vi "load RT config file.vi"(11 "configuration file path (RT local)":path) -> (0 "error out":errorcluster, 1 "unmatched parameters":string[](array[string]), 2 "Default parameters":string[](array[string]), 3 "config data out":T18={"Message"={"Parameters"={"FPGA Ref"=refnum, "configID"=0, "activeChannels"=[]}, "Variables"={"RT Status"={"Comms loop"=FALSE, "scheduler loop"=FALSE, "data process loop"=FALSE, "FIFO loop"=FALSE, "Command Stream"=FALSE, "Error Stream"=FALSE, "FPGA FIFO"=FALSE, "Data Stream"=FALSE}, "watchdog"=timestamp(0 s since 1904-01-01), "limitsEnabled"=FALSE, "Interlocks"={"gearboxOil"=FALSE, "bearingOil"=FALSE, "gearboxAir"=FALSE}}}, "FIFO"={"Params"={"FPGA ref"=refnum, "Total Channels"=0}, "Variables"={"FIFO wait counter"=0, "FIFO read trigger"=0}}, "Comms data"={"Parameters"={"error writer name"="", "command reader name"="", "error buffer size"=0, "command buffer size"=0, "scanivalveIP"="", "scanivalvePeriod"=0}, "Variables"={"listen schedule"=0, "incident buffer"=[], "command stream"="", "error stream"="", "waiting for command stream connect"=FALSE, "waiting for error stream connect"=FALSE, "scanivalve connection"=refnum, "scanivalveScheduleID"=0, "activeScanivalvePorts"=[], "channelCount"=0}, "scanivalveConfig"={"listS"={"period"=0, "ADtrig"=FALSE, "ScanTrig"=FALSE, "page"=0, "qpkts"=0}, "listC"={"ZC"=FALSE, "unitScan"="", "CvtUnit"=0.0, "bin"=FALSE, "EU"=FALSE}, "listSG"={"Avg1"=0, "FPS1"=0, "SGEnable1"=FALSE}, "activeChannels"={"Chan1"={"101"=FALSE, "102"=FALSE, "103"=FALSE, "104"=FALSE, "109"=FALSE, "110"=FALSE, "111"=FALSE, "112"=FALSE, "201"=FALSE, "202"=FALSE, "203"=FALSE, "204"=FALSE, "209"=FALSE, "210"=FALSE, "211"=FALSE, "212"=FALSE, "301"=FALSE, "302"=FALSE, "303"=FALSE, "304"=FALSE, "309"=FALSE, "310"=FALSE, "311"=FALSE, "312"=FALSE, "401"=FALSE, "402"=FALSE, "403"=FALSE, "404"=FALSE, "409"=FALSE, "410"=FALSE, "411"=FALSE, "412"=FALSE}}}}, "Data processor"={"Parameters"={"FPGA Ref"=refnum, "data stream"={"data writer name"="error writer", "NS write buffer size"=16, "NS Buffer length"=0}, "FIFO Depth"=0, "Channel controls"={"FIFO channel count"=0, "active indices"=[], "active channels"=0, "channelScaling"=[], "scanivalveCount"=0, "channels"=[]}, "safetyChannels"={"oilP"=0, "airP"=0, "water"=0, "channelLimits"=[]}, "speedChannel"=0, "maxSpeedLimit"=0.0, "Torque"={"fixedOffset"=0.0, "filter"=FALSE, "fallingEdge"=FALSE, "swapEncoders"=FALSE}}, "Variables"={"Intermediary buffer"=[], "buffer position"=0, "write loop counter"=0, "NS write trigger"=0, "NS Connection status"=FALSE, "waiting for NS"=FALSE, "labAmbient"={"pressure"=0.0, "temperature"=0.0}, "scanivalvePorts"=[], "scanivalvePressures"=[], "data stream"="", "activeChannelLimitIndex"=[], "runningSpeedLimit"=0.0, "speedChannelIndex"=0, "Interlocks"={"gearboxOil"=FALSE, "bearingOil"=FALSE, "gearboxAir"=FALSE}, "interlockChannels"={"gearboxOil"=0, "bearingOil"=0, "air"=0}, "limitStates"=[]}}})   [LabVIEW 2018]
uses:
  RT/Type Defs/Message loop data.ctl
  RT/Type Defs/FPGA reference.ctl
  RT/Type Defs/RT Status.ctl
  RT/Type Defs/Analogue loop data.ctl
  RT/Communications loop/comms data.ctl
  RT/Type Defs/generic incident.ctl
  ICL-LabVIEW_General/Scanivalve API project/full interface/polymorphic/scanivalveConfig.ctl
  ICL-LabVIEW_General/Scanivalve API project/full interface/listS.ctl
  ICL-LabVIEW_General/Scanivalve API project/full interface/listC.ctl
  ICL-LabVIEW_General/Scanivalve API project/full interface/listSG.ctl
  ICL-LabVIEW_General/Scanivalve API project/full interface/chan1.ctl
  RT/Type Defs/Data processing loop data.ctl
  type defs/channelControl.ctl
  RT/Type Defs/channelScalingTypes.ctl
  RT/Type Defs/scalingMethods.ctl
  ICL-LabVIEW_General/data channels/parent class/Data Channel.lvclass
  type defs/channelLimitControl.ctl
  type defs/limitActions.ctl
  RT/Type Defs/configFilePath.ctl
  <vilib>/Utility/config.llb/Read Key (U32).vi
  <vilib>/Utility/config.llb/Read Key (String).vi
  <vilib>/Utility/config.llb/Read Key (I32).vi
  <vilib>/Utility/config.llb/Read Key (Double).vi
  <vilib>/Utility/config.llb/Read Key (Boolean).vi
  <vilib>/Utility/config.llb/NI_LVConfig.lvlib
  ICL-LabVIEW_General/Scanivalve API project/Scanivalve API.lvlib
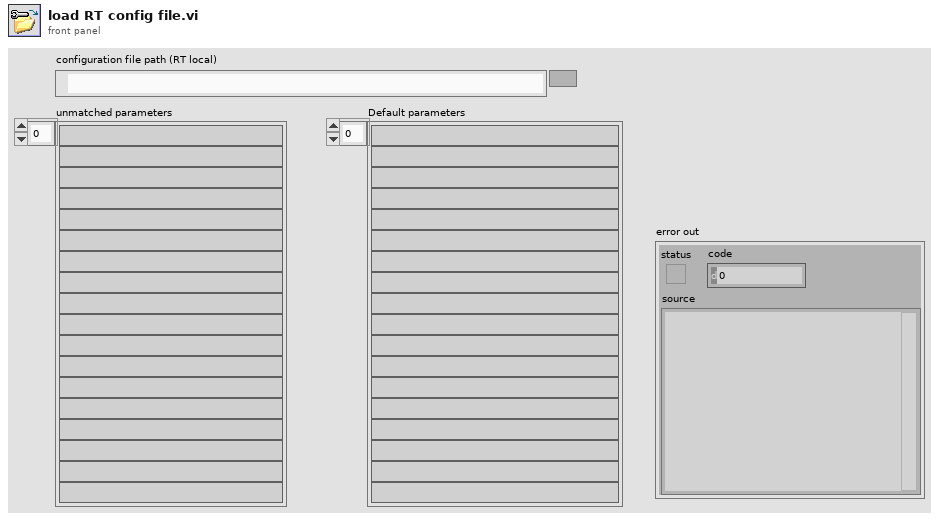
[diagram p1: front panel]
types:
  T1 = typedef "Message loop data.ctl" = cluster{"Parameters":cluster{"FPGA Ref":T2, "configID":u32, "activeChannels":cluster{"index":u16, "name":string}[]}, "Variables":cluster{"RT Status":T3, "watchdog":timestamp, "limitsEnabled":bool, "Interlocks":cluster{"gearboxOil":bool, "bearingOil":bool, "gearboxAir":bool}}}
  T2 = typedef "FPGA reference.ctl" = refnum<k20>
  T3 = typedef "RT Status.ctl" = cluster{"Comms loop":bool, "scheduler loop":bool, "data process loop":bool, "FIFO loop":bool, "Command Stream":bool, "Error Stream":bool, "FPGA FIFO":bool, "Data Stream":bool}
  T4 = typedef "Analogue loop data.ctl" = cluster{"Params":cluster{"FPGA ref":T2, "Total Channels":u32}, "Variables":cluster{"FIFO wait counter":u16, "FIFO read trigger":u32}}
  T5 = typedef "comms data.ctl" = cluster{"Parameters":cluster{"error writer name":string, "command reader name":string, "error buffer size":i32, "command buffer size":i32, "scanivalveIP":string, "scanivalvePeriod":u16}, "Variables":cluster{"listen schedule":u32, "incident buffer":T6[], "command stream":refnum<k21>, "error stream":refnum<k21>, "waiting for command stream connect":bool, "waiting for error stream connect":bool, "scanivalve connection":refnum<k5>, "scanivalveScheduleID":u32, "activeScanivalvePorts":i32[], "channelCount":i16}, "scanivalveConfig":T7}
  T6 = typedef "generic incident.ctl" = cluster{"timestamp":timestamp, "type":string, "Variant":variant}
  T7 = typedef "Scanivalve API.lvlib/scanivalveConfig.ctl" = cluster{"listS":T8, "listC":T9, "listSG":T10, "activeChannels":T11}
  T8 = typedef "Scanivalve API.lvlib/listS.ctl" = cluster{"period":u16, "ADtrig":bool, "ScanTrig":bool, "page":u16, "qpkts":u16}
  T9 = typedef "Scanivalve API.lvlib/listC.ctl" = cluster{"ZC":bool, "unitScan":string, "CvtUnit":dbl, "bin":bool, "EU":bool}
  T10 = typedef "Scanivalve API.lvlib/listSG.ctl" = cluster{"Avg1":u16, "FPS1":u16, "SGEnable1":bool}
  T11 = typedef "Scanivalve API.lvlib/chan1.ctl" = cluster{"Chan1":cluster{"101":bool, "102":bool, "103":bool, "104":bool, "109":bool, "110":bool, "111":bool, "112":bool, "201":bool, "202":bool, "203":bool, "204":bool, "209":bool, "210":bool, "211":bool, "212":bool, "301":bool, "302":bool, "303":bool, "304":bool, "309":bool, "310":bool, "311":bool, "312":bool, "401":bool, "402":bool, "403":bool, "404":bool, "409":bool, "410":bool, "411":bool, "412":bool}}
  T12 = typedef "Data processing loop data.ctl" = cluster{"Parameters":cluster{"FPGA Ref":T2, "data stream":cluster{"data writer name":string, "NS write buffer size":i32, "NS Buffer length":u32}, "FIFO Depth":u32, "Channel controls":cluster{"FIFO channel count":i32, "active indices":i16[], "active channels":i32, "channelScaling":T13[], "scanivalveCount":i32, "channels":refnum<class "Data Channel.lvclass">[]}, "safetyChannels":cluster{"oilP":u16, "airP":u16, "water":u16, "channelLimits":T16[]}, "speedChannel":i32, "maxSpeedLimit":dbl, "Torque":cluster{"fixedOffset":dbl, "filter":bool, "fallingEdge":bool, "swapEncoders":bool}}, "Variables":cluster{"Intermediary buffer":dbl[][], "buffer position":u32, "write loop counter":u16, "NS write trigger":u32, "NS Connection status":bool, "waiting for NS":bool, "labAmbient":cluster{"pressure":dbl, "temperature":dbl}, "scanivalvePorts":u16[], "scanivalvePressures":dbl[], "data stream":refnum<k21>, "activeChannelLimitIndex":u16[], "runningSpeedLimit":dbl, "speedChannelIndex":i32, "Interlocks":cluster{"gearboxOil":bool, "bearingOil":bool, "gearboxAir":bool}, "interlockChannels":cluster{"gearboxOil":i32, "bearingOil":i32, "air":i32}, "limitStates":cluster{"warn":bool, "alarm":bool}[]}}
  T13 = typedef "channelControl.ctl" = cluster{"index":u16, "active":bool, "channelType":T14, "module":u16, "terminal":u16, "channelName":string, "scalingMethod":T15, "scalingParameters":dbl[], "scaledUnits":string, "tempOffset":dbl}
  T14 = typedef "channelScalingTypes.ctl" = enum16{"calculation", "measurement", "scanivalve", "output", "digital"}
  T15 = typedef "scalingMethods.ctl" = enum16{"none", "linear", "thermocouple", "polynomial", "encoder", "RTD"}
  T16 = typedef "channelLimitControl.ctl" = cluster{"channelID":u16, "Enabled":bool, "warnValue":dbl, "limitValue":dbl, "Invert":bool, "limitAction":T17}
  T17 = typedef "limitActions.ctl" = enum16{"stop", "shutdown", "ignore"}
  T18 = cluster{"Message":T1, "FIFO":T4, "Comms data":T5, "Data processor":T12}
  T19 = typedef "configFilePath.ctl" = path
  T20 = typedef "NI_LVConfig.lvlib/Config Data RefNum.ctl" = refnum<k1>
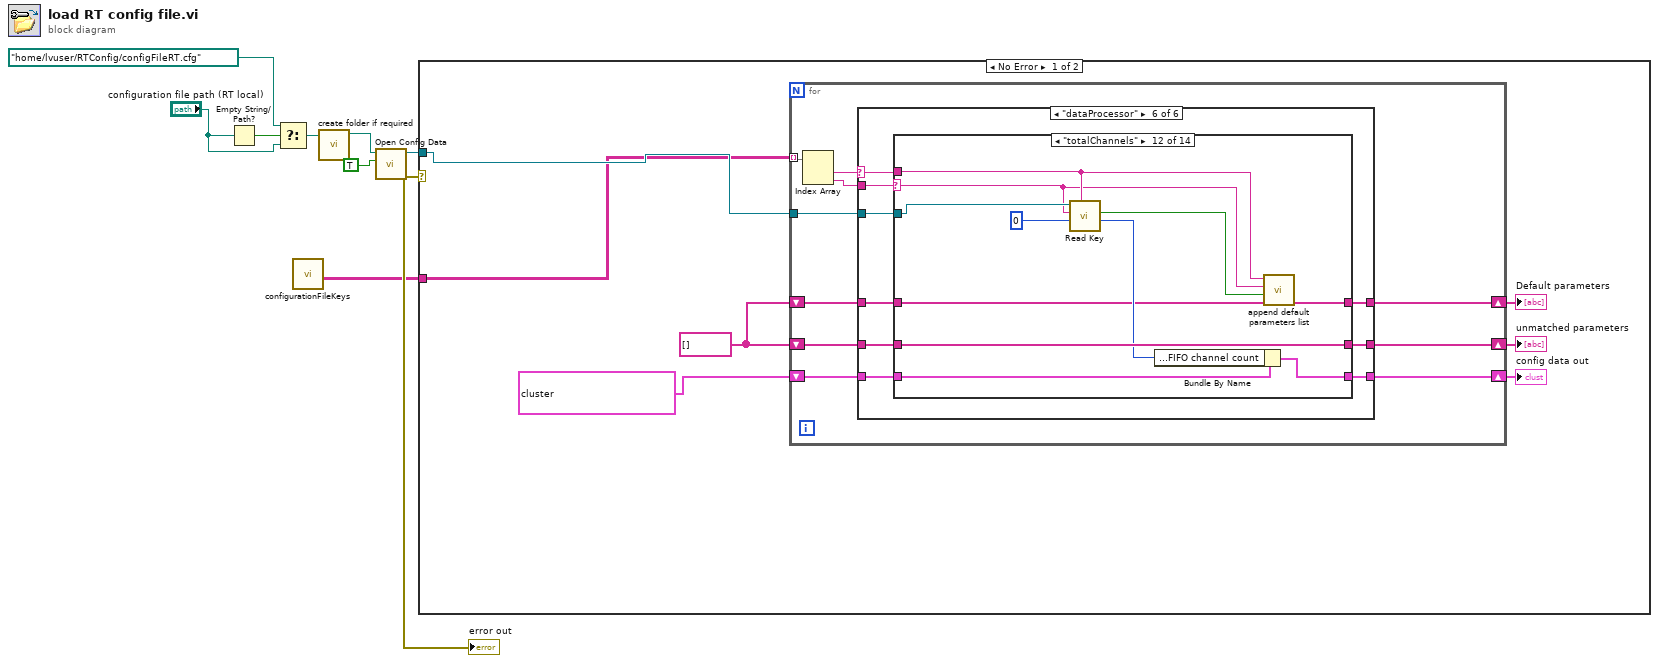
[diagram p0: block diagram]
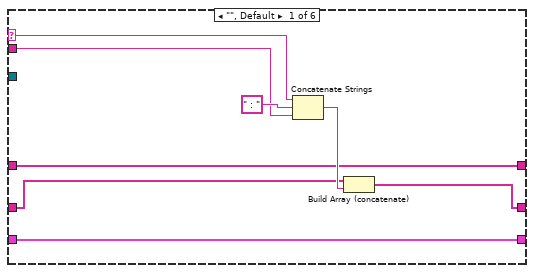
[diagram p2: hidden frame]
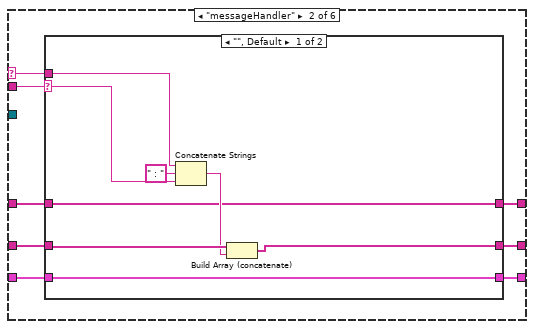
[diagram p3: hidden frame]
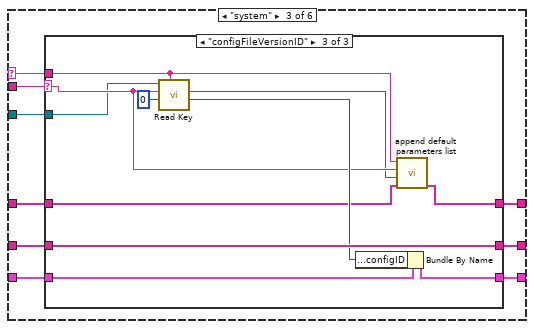
[diagram p5: hidden frame]
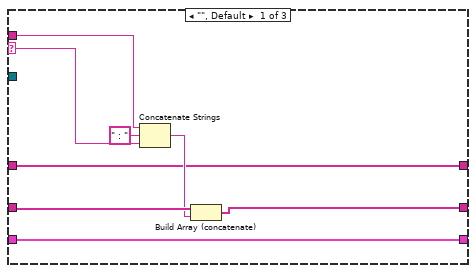
[diagram p6: hidden frame]
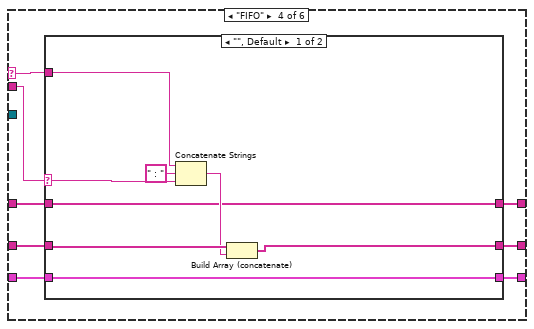
[diagram p8: hidden frame]
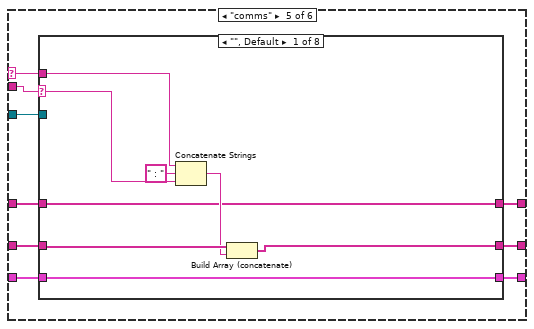
[diagram p10: hidden frame]
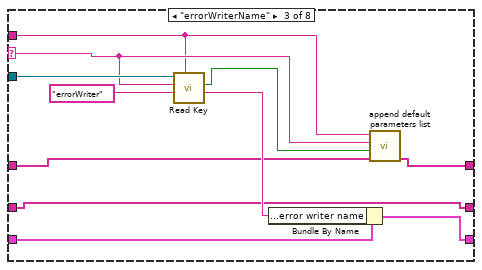
[diagram p12: hidden frame]
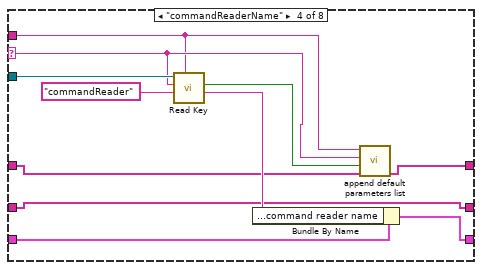
[diagram p13: hidden frame]
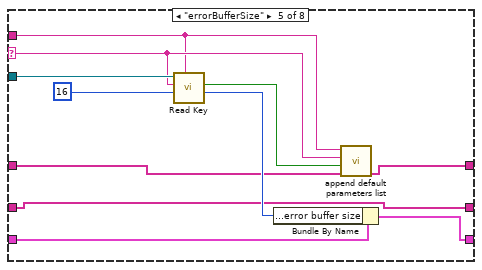
[diagram p14: hidden frame]
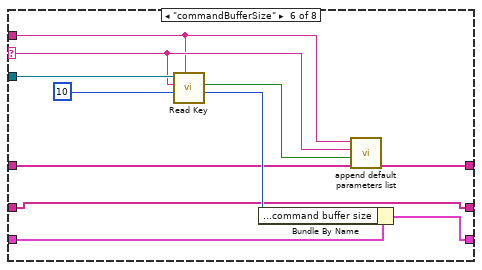
[diagram p15: hidden frame]
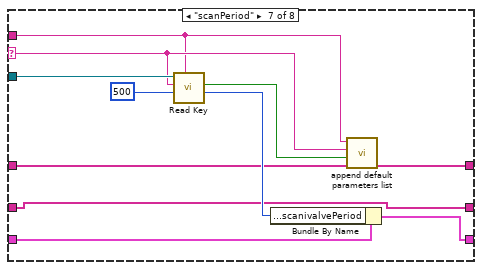
[diagram p16: hidden frame]
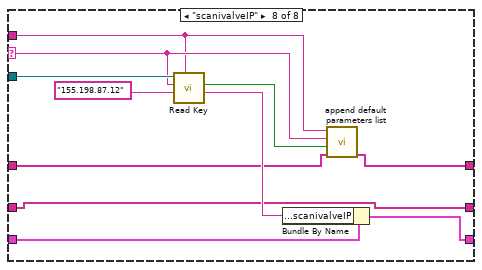
[diagram p17: hidden frame]
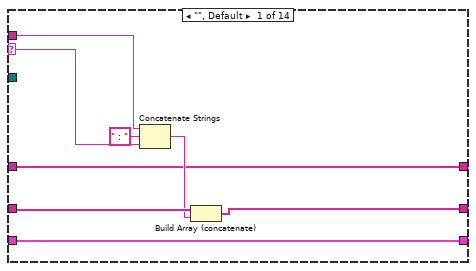
[diagram p18: hidden frame]
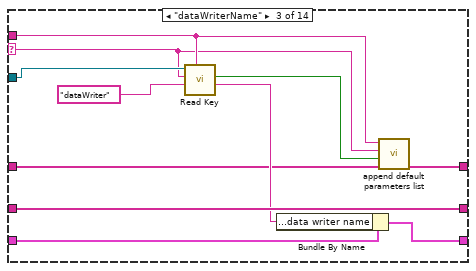
[diagram p20: hidden frame]
diagram:
  n1 = Empty String/Path?(string/path="configuration file path (RT local)") -> (empty?=w6:bool)
  n2 = Select(t=T19 path "/home/lvuser/RTConfig/configFileRT.cfg" ("file path (use dialog)"), s=w6, f="configuration file path (RT local)") -> (s? t:f=w2:T19)
  n3 = call "configurationFileKeys.vi"() -> ("configKeysRT"=w4:string[][])  [unwired: 9 in, 2 out]
  n4 = call "create folder if required.vi"("folder path"=w2) -> ("actual path"=w1:path)  [unwired: 9 in, 1 out]
  n5 = call <vilib>:"Open Config Data.vi"("create file if necessary (T)"=TRUE, "configuration file path"=w1) -> ("error out"=w7:errorcluster, "refnum"=w9:T20)  [unwired: 7 in, 1 out]
  "error out" <- w7
  n6 = case shown="No Error" w7 {
    tunnel: w9 -> [w14 _]
    tunnel: w4 -> [w13 _]
    frame No Error {
      w12 = string[] []
      n7 = for {
        shift-right: [w25] -> w16
        shift-left: w12 -> [w26]
        shift-right: [w23] -> w10
        shift-left: T18 {"Message"={"Parameters"={"FPGA Ref"=refnum, "configID"=0, "activeChannels"=[]}, "Variables"={"RT Status"={"Comms loop"=FALSE, "scheduler loop"=FALSE, "data process loop"=FALSE, "FIFO loop"=FALSE, "Command Stream"=FALSE, "Error Stream"=FALSE, "FPGA FIFO"=FALSE, "Data Stream"=FALSE}, "watchdog"=timestamp(0 s since 1904-01-01), "limitsEnabled"=FALSE, "Interlocks"={"gearboxOil"=FALSE, "bearingOil"=FALSE, "gearboxAir"=FALSE}}}, "FIFO"={"Params"={"FPGA ref"=refnum, "Total Channels"=0}, "Variables"={"FIFO wait counter"=0, "FIFO read trigger"=0}}, "Comms data"={"Parameters"={"error writer name"="error writer", "command reader name"="command reader", "error buffer size"=16, "command buffer size"=16, "scanivalveIP"="", "scanivalvePeriod"=16}, "Variables"={"listen schedule"=0, "incident buffer"=[], "command stream"="", "error stream"="", "waiting for command stream connect"=FALSE, "waiting for error stream connect"=FALSE, "scanivalve connection"=refnum, "scanivalveScheduleID"=16, "activeScanivalvePorts"=[], "channelCount"=0}, "scanivalveConfig"={"listS"={"period"=0, "ADtrig"=FALSE, "ScanTrig"=FALSE, "page"=0, "qpkts"=0}, "listC"={"ZC"=FALSE, "unitScan"="", "CvtUnit"=0.0, "bin"=FALSE, "EU"=FALSE}, "listSG"={"Avg1"=0, "FPS1"=0, "SGEnable1"=FALSE}, "activeChannels"={"Chan1"={"101"=FALSE, "102"=FALSE, "103"=FALSE, "104"=FALSE, "109"=FALSE, "110"=FALSE, "111"=FALSE, "112"=FALSE, "201"=FALSE, "202"=FALSE, "203"=FALSE, "204"=FALSE, "209"=FALSE, "210"=FALSE, "211"=FALSE, "212"=FALSE, "301"=FALSE, "302"=FALSE, "303"=FALSE, "304"=FALSE, "309"=FALSE, "310"=FALSE, "311"=FALSE, "312"=FALSE, "401"=FALSE, "402"=FALSE, "403"=FALSE, "404"=FALSE, "409"=FALSE, "410"=FALSE, "411"=FALSE, "412"=FALSE}}}}, "Data processor"={"Parameters"={"FPGA Ref"=refnum, "data stream"={"data writer name"="", "NS write buffer size"=0, "NS Buffer length"=0}, "FIFO Depth"=0, "Channel controls"={"FIFO channel count"=0, "active indices"=[], "active channels"=0, "channelScaling"=[], "scanivalveCount"=0, "channels"=[]}, "safetyChannels"={"oilP"=0, "airP"=0, "water"=0, "channelLimits"=[]}, "speedChannel"=0, "maxSpeedLimit"=0.0, "Torque"={"fixedOffset"=0.0, "filter"=FALSE, "fallingEdge"=FALSE, "swapEncoders"=FALSE}}, "Variables"={"Intermediary buffer"=[], "buffer position"=0, "write loop counter"=0, "NS write trigger"=0, "NS Connection status"=FALSE, "waiting for NS"=FALSE, "labAmbient"={"pressure"=0.0, "temperature"=0.0}, "scanivalvePorts"=[], "scanivalvePressures"=[], "data stream"="", "activeChannelLimitIndex"=[], "runningSpeedLimit"=0.0, "speedChannelIndex"=0, "Interlocks"={"gearboxOil"=FALSE, "bearingOil"=FALSE, "gearboxAir"=FALSE}, "interlockChannels"={"gearboxOil"=0, "bearingOil"=0, "air"=0}, "limitStates"=[]}}} ("config data 2") -> [w24]
        tunnel: w14 -> [w22]
        tunnel: w13 -> [w21] mode=indexing
        shift-right: [w18] -> w11
        shift-left: w12 -> [w17]
        n8 = Index Array(array=w21) -> (element #1=w20:string, element #2=w19:string)  [unwired: 2 in]
        n9 = case shown="\"dataProcessor\"" w20 {
          selector: w20 -> [w30 w41 w61 w91 w111 w197]
          tunnel: w26 -> [w32 w42 w62 w92 w112 w198]
          tunnel: [w31 w40 w60 w90 w110 w196] -> w25
          tunnel: w24 -> [w29 w38 w58 w88 w109 w194]
          tunnel: [w29 w39 w59 w89 w108 w195] -> w23
          tunnel: w22 -> [_ _ w54 _ w107 w193]
          tunnel: w19 -> [w28 w37 w57 w87 w106 w192]
          tunnel: [w27 w36 w56 w86 w104 w191] -> w18
          tunnel: w17 -> [w27 w35 w55 w85 w105 w190]
          frame "", Default {
            n10 = Concatenate Strings(w30, " : " ("string"), w28) -> (w33:string)
            n11 = Build Array (concatenate)(w32, w33) -> (w31:string[])
          }
          frame "messageHandler" {
            n12 = case shown="\"\", Default" w37 {
              selector: w37 -> [w48 _]
              tunnel: w42 -> [w50 w53]
              tunnel: w41 -> [w49 _]
              tunnel: [w45 w53] -> w40
              tunnel: [w44 w52] -> w39
              tunnel: w38 -> [w44 w52]
              tunnel: [w43 w51] -> w36
              tunnel: w35 -> [w43 w51]
              frame "", Default {
                n13 = Concatenate Strings(w49, " : " ("string"), w48) -> (w46:string)
                n14 = Build Array (concatenate)(w50, w46) -> (w45:string[])
              }
              frame "none" {
              }
            }
          }
          frame "system" {
            n15 = case shown="\"configFileVersionID\"" w57 {
              selector: w57 -> [w68 _ w76]
              tunnel: w62 -> [w70 w73 w84]
              tunnel: w61 -> [w69 _ w77]
              tunnel: [w65 w73 w84] -> w60
              tunnel: [w64 w72 w81] -> w59
              tunnel: w58 -> [w64 w72 w83]
              tunnel: [w63 w71 w78] -> w56
              tunnel: w55 -> [w63 w71 w79]
              tunnel: w54 -> [_ _ w74]
              frame "", Default {
                n16 = Concatenate Strings(w69, " : " ("string"), w68) -> (w66:string)
                n17 = Build Array (concatenate)(w70, w66) -> (w65:string[])
              }
              frame "none" {
              }
              frame "configFileVersionID" {
                n18 = call-poly <vilib>:"Read Key.vi"("section"=w77, "default value"=u32 0, "key"=w76, "refnum"=w74) -> ("value"=w80:u32, "found?"=w75:bool)  [unwired: 4 in, 2 out]
                n19 = Bundle By Name(cluster=w83, "Message.Parameters.configID"=w80) -> (w81:T18)
                n20 = call "append default parameters list.vi"("default parameters in"=w79, "parameter found?"=w75, "Key"=w76, "Section"=w77) -> ("default parameters out"=w78:string[])  [unwired: 7 in]
              }
            }
          }
          frame "FIFO" {
            n21 = case shown="\"\", Default" w87 {
              selector: w87 -> [w98 _]
              tunnel: w92 -> [w100 w103]
              tunnel: w91 -> [w99 _]
              tunnel: [w95 w103] -> w90
              tunnel: [w94 w102] -> w89
              tunnel: w88 -> [w94 w102]
              tunnel: [w93 w101] -> w86
              tunnel: w85 -> [w93 w101]
              frame "", Default {
                n22 = Concatenate Strings(w99, " : " ("string"), w98) -> (w96:string)
                n23 = Build Array (concatenate)(w100, w96) -> (w95:string[])
              }
              frame "none" {
              }
            }
          }
          frame "comms" {
            n24 = case shown="\"\", Default" w106 {
              selector: w106 -> [w118 _ w125 w136 w149 w158 w169 w180]
              tunnel: w112 -> [w120 w123 w129 w140 w151 w162 w173 w184]
              tunnel: w111 -> [w119 _ w124 w135 w148 w157 w168 w179]
              tunnel: [w115 w123 w129 w140 w151 w162 w173 w184] -> w110
              tunnel: w109 -> [w114 w122 w132 w143 w155 w166 w177 w188]
              tunnel: [w114 w122 w131 w142 w154 w165 w176 w187] -> w108
              tunnel: w107 -> [_ _ w134 w145 w156 w167 w178 w189]
              tunnel: w105 -> [w113 w121 w128 w139 w147 w161 w172 w183]
              tunnel: [w113 w121 w127 w138 w146 w160 w171 w182] -> w104
              frame "", Default {
                n25 = Concatenate Strings(w119, " : " ("string"), w118) -> (w116:string)
                n26 = Build Array (concatenate)(w120, w116) -> (w115:string[])
              }
              frame "none" {
              }
              frame "errorWriterName" {
                n27 = call-poly <vilib>:"Read Key.vi"("section"=w124, "default value"="errorWriter" ("Parameters.error writer name"), "key"=w125, "refnum"=w134) -> ("value"=w130:string, "found?"=w126:bool)  [unwired: 4 in, 2 out]
                n28 = Bundle By Name(cluster=w132, "Comms data.Parameters.error writer name"=w130) -> (w131:T18)
                n29 = call "append default parameters list.vi"("default parameters in"=w128, "parameter found?"=w126, "Key"=w125, "Section"=w124) -> ("default parameters out"=w127:string[])  [unwired: 7 in]
              }
              frame "commandReaderName" {
                n30 = call-poly <vilib>:"Read Key.vi"("section"=w135, "default value"="commandReader" ("Parameters.error writer name"), "key"=w136, "refnum"=w145) -> ("value"=w141:string, "found?"=w137:bool)  [unwired: 4 in, 2 out]
                n31 = Bundle By Name(cluster=w143, "Comms data.Parameters.command reader name"=w141) -> (w142:T18)
                n32 = call "append default parameters list.vi"("default parameters in"=w139, "parameter found?"=w137, "Key"=w136, "Section"=w135) -> ("default parameters out"=w138:string[])  [unwired: 7 in]
              }
              frame "errorBufferSize" {
                n33 = call-poly <vilib>:"Read Key.vi"("section"=w148, "default value"=16 ("Parameters.error buffer size"), "key"=w149, "refnum"=w156) -> ("value"=w153:i32, "found?"=w150:bool)  [unwired: 4 in, 2 out]
                n34 = Bundle By Name(cluster=w155, "Comms data.Parameters.error buffer size"=w153) -> (w154:T18)
                n35 = call "append default parameters list.vi"("default parameters in"=w147, "parameter found?"=w150, "Key"=w149, "Section"=w148) -> ("default parameters out"=w146:string[])  [unwired: 7 in]
              }
              frame "commandBufferSize" {
                n36 = call-poly <vilib>:"Read Key.vi"("section"=w157, "default value"=10 ("Parameters.error buffer size"), "key"=w158, "refnum"=w167) -> ("value"=w164:i32, "found?"=w159:bool)  [unwired: 4 in, 2 out]
                n37 = Bundle By Name(cluster=w166, "Comms data.Parameters.command buffer size"=w164) -> (w165:T18)
                n38 = call "append default parameters list.vi"("default parameters in"=w161, "parameter found?"=w159, "Key"=w158, "Section"=w157) -> ("default parameters out"=w160:string[])  [unwired: 7 in]
              }
              frame "scanPeriod" {
                n39 = call-poly <vilib>:"Read Key.vi"("section"=w168, "default value"=500 ("Parameters.error buffer size"), "key"=w169, "refnum"=w178) -> ("value"=w175:i32, "found?"=w170:bool)  [unwired: 4 in, 2 out]
                n40 = Bundle By Name(cluster=w177, "Comms data.Parameters.scanivalvePeriod"=w175) -> (w176:T18)
                n41 = call "append default parameters list.vi"("default parameters in"=w172, "parameter found?"=w170, "Key"=w169, "Section"=w168) -> ("default parameters out"=w171:string[])  [unwired: 7 in]
              }
              frame "scanivalveIP" {
                n42 = call-poly <vilib>:"Read Key.vi"("section"=w179, "default value"="155.198.87.12" ("Parameters.scanivalveIP"), "key"=w180, "refnum"=w189) -> ("value"=w186:string, "found?"=w181:bool)  [unwired: 4 in, 2 out]
                n43 = Bundle By Name(cluster=w188, "Comms data.Parameters.scanivalveIP"=w186) -> (w187:T18)
                n44 = call "append default parameters list.vi"("default parameters in"=w183, "parameter found?"=w181, "Key"=w180, "Section"=w179) -> ("default parameters out"=w182:string[])  [unwired: 7 in]
              }
            }
          }
          frame "dataProcessor" {
            n45 = case shown="\"totalChannels\"" w192 {
              selector: w192 -> [w204 _ w211 w222 w233 w244 w255 w267 w278 w289 w300 w311 w322 _]
              tunnel: w198 -> [w206 w209 w220 w231 w242 w253 w264 w275 w286 w297 w308 w319 w330 w334]
              tunnel: w197 -> [w205 _ w212 w223 w234 w245 w256 w268 w279 w290 w301 w312 w323 _]
              tunnel: [w201 w209 w220 w231 w242 w253 w264 w275 w286 w297 w308 w319 w330 w334] -> w196
              tunnel: [w200 w208 w218 w229 w240 w251 w262 w273 w284 w295 w306 w317 w328 w331] -> w195
              tunnel: w194 -> [w200 w208 w219 w230 w241 w252 w263 w274 w285 w296 w307 w318 w329 w332]
              tunnel: w193 -> [_ _ w215 w226 w237 w248 w259 w271 w282 w293 w304 w315 w326 w333]
              tunnel: [w199 w207 w214 w225 w236 w247 w258 w270 w281 w292 w303 w314 w325 w335] -> w191
              tunnel: w190 -> [w199 w207 w213 w224 w235 w246 w257 w269 w280 w291 w302 w313 w324 w335]
              frame "", Default {
                n46 = Concatenate Strings(w205, " : " ("string"), w204) -> (w202:string)
                n47 = Build Array (concatenate)(w206, w202) -> (w201:string[])
              }
              frame "none" {
              }
              frame "dataWriterName" {
                n48 = call-poly <vilib>:"Read Key.vi"("section"=w212, "default value"="dataWriter", "key"=w211, "refnum"=w215) -> ("value"=w216:string, "found?"=w210:bool)  [unwired: 4 in, 2 out]
                n49 = Bundle By Name(cluster=w219, "Data processor.Parameters.data stream.data writer name"=w216) -> (w218:T18)
                n50 = call "append default parameters list.vi"("default parameters in"=w213, "parameter found?"=w210, "Key"=w211, "Section"=w212) -> ("default parameters out"=w214:string[])  [unwired: 7 in]
              }
              frame "encoderOffset" {
                n51 = call-poly <vilib>:"Read Key.vi"("section"=w223, "default value"=0.0, "key"=w222, "refnum"=w226) -> ("value"=w227:dbl, "found?"=w221:bool)  [unwired: 4 in, 2 out]
                n52 = Bundle By Name(cluster=w230, "Data processor.Parameters.Torque.fixedOffset"=w227) -> (w229:T18)
                n53 = call "append default parameters list.vi"("default parameters in"=w224, "parameter found?"=w221, "Key"=w222, "Section"=w223) -> ("default parameters out"=w225:string[])  [unwired: 7 in]
              }
              frame "filter" {
                n54 = call-poly <vilib>:"Read Key.vi"("section"=w234, "default value"=TRUE, "key"=w233, "refnum"=w237) -> ("value"=w238:bool, "found?"=w232:bool)  [unwired: 4 in, 2 out]
                n55 = Bundle By Name(cluster=w241, "Data processor.Parameters.Torque.filter"=w238) -> (w240:T18)
                n56 = call "append default parameters list.vi"("default parameters in"=w235, "parameter found?"=w232, "Key"=w233, "Section"=w234) -> ("default parameters out"=w236:string[])  [unwired: 7 in]
              }
              frame "fallingEdge" {
                n57 = call-poly <vilib>:"Read Key.vi"("section"=w245, "default value"=TRUE, "key"=w244, "refnum"=w248) -> ("value"=w249:bool, "found?"=w243:bool)  [unwired: 4 in, 2 out]
                n58 = Bundle By Name(cluster=w252, "Data processor.Parameters.Torque.fallingEdge"=w249) -> (w251:T18)
                n59 = call "append default parameters list.vi"("default parameters in"=w246, "parameter found?"=w243, "Key"=w244, "Section"=w245) -> ("default parameters out"=w247:string[])  [unwired: 7 in]
              }
              frame "swapEncoders" {
                n60 = call-poly <vilib>:"Read Key.vi"("section"=w256, "default value"=TRUE, "key"=w255, "refnum"=w259) -> ("value"=w260:bool, "found?"=w254:bool)  [unwired: 4 in, 2 out]
                n61 = Bundle By Name(cluster=w263, "Data processor.Parameters.Torque.swapEncoders"=w260) -> (w262:T18)
                n62 = call "append default parameters list.vi"("default parameters in"=w257, "parameter found?"=w254, "Key"=w255, "Section"=w256) -> ("default parameters out"=w258:string[])  [unwired: 7 in]
              }
              frame "NetStreamWriteBufferSize" {
                n63 = call-poly <vilib>:"Read Key.vi"("section"=w268, "default value"=10, "key"=w267, "refnum"=w271) -> ("value"=w272:i32, "found?"=w266:bool)  [unwired: 4 in, 2 out]
                n64 = Bundle By Name(cluster=w274, "Data processor.Parameters.data stream.NS write buffer size"=w272) -> (w273:T18)
                n65 = call "append default parameters list.vi"("default parameters in"=w269, "parameter found?"=w266, "Key"=w267, "Section"=w268) -> ("default parameters out"=w270:string[])  [unwired: 7 in]
              }
              frame "NetStreamBufferLength" {
                n66 = call-poly <vilib>:"Read Key.vi"("section"=w279, "default value"=50000, "key"=w278, "refnum"=w282) -> ("value"=w283:i32, "found?"=w277:bool)  [unwired: 4 in, 2 out]
                n67 = Bundle By Name(cluster=w285, "Data processor.Parameters.data stream.NS Buffer length"=w283) -> (w284:T18)
                n68 = call "append default parameters list.vi"("default parameters in"=w280, "parameter found?"=w277, "Key"=w278, "Section"=w279) -> ("default parameters out"=w281:string[])  [unwired: 7 in]
              }
              frame "speedChannel" {
                n69 = call-poly <vilib>:"Read Key.vi"("section"=w290, "default value"=0, "key"=w289, "refnum"=w293) -> ("value"=w294:i32, "found?"=w288:bool)  [unwired: 4 in, 2 out]
                n70 = Bundle By Name(cluster=w296, "Data processor.Parameters.speedChannel"=w294) -> (w295:T18)
                n71 = call "append default parameters list.vi"("default parameters in"=w291, "parameter found?"=w288, "Key"=w289, "Section"=w290) -> ("default parameters out"=w292:string[])  [unwired: 7 in]
              }
              frame "oilPressureChannel" {
                n72 = call-poly <vilib>:"Read Key.vi"("section"=w301, "default value"=0, "key"=w300, "refnum"=w304) -> ("value"=w305:i32, "found?"=w299:bool)  [unwired: 4 in, 2 out]
                n73 = Bundle By Name(cluster=w307, "Data processor.Parameters.safetyChannels.oilP"=w305) -> (w306:T18)
                n74 = call "append default parameters list.vi"("default parameters in"=w302, "parameter found?"=w299, "Key"=w300, "Section"=w301) -> ("default parameters out"=w303:string[])  [unwired: 7 in]
              }
              frame "totalChannels" {
                n75 = call-poly <vilib>:"Read Key.vi"("section"=w312, "default value"=0, "key"=w311, "refnum"=w315) -> ("value"=w316:i32, "found?"=w310:bool)  [unwired: 4 in, 2 out]
                n76 = Bundle By Name(cluster=w318, "Data processor.Parameters.Channel controls.FIFO channel count"=w316) -> (w317:T18)
                n77 = call "append default parameters list.vi"("default parameters in"=w313, "parameter found?"=w310, "Key"=w311, "Section"=w312) -> ("default parameters out"=w314:string[])  [unwired: 7 in]
              }
              frame "maxSpeedLimit" {
                n78 = call-poly <vilib>:"Read Key.vi"("section"=w323, "default value"=1030.0, "key"=w322, "refnum"=w326) -> ("value"=w327:dbl, "found?"=w321:bool)  [unwired: 4 in, 2 out]
                n79 = Bundle By Name(cluster=w329, "Data processor.Parameters.maxSpeedLimit"=w327) -> (w328:T18)
                n80 = call "append default parameters list.vi"("default parameters in"=w324, "parameter found?"=w321, "Key"=w322, "Section"=w323) -> ("default parameters out"=w325:string[])  [unwired: 7 in]
              }
              frame "limitChannels" {
                n81 = call "read channel limits config.vi"("config data in"=w332, "configFile ref"=w333) -> ("config data out"=w331:T18)  [unwired: 9 in]
              }
            }
          }
        }
      }
      "unmatched parameters" <- w16
      "Default parameters" <- w11
      "config data out" <- w10
    }
    frame Error {
    }
  }
